vi "ULx Clear Task.vi"(0 "task in":refnum<k24>, 11 "error in":errorcluster) -> (15 "error out":errorcluster)   [LabVIEW 2020]
doc: "Clears the task. Before clearing, this VI stops the task, if necessary, and releases any resources the task reserved. You cannot use a task after you clear it unless you recreate the task."
uses:
  C:/Users/William/Documents/LV 2020 builds/LeaktestDAQ/Source-v33/ULx_LV.dll
  ULx_LV.dll
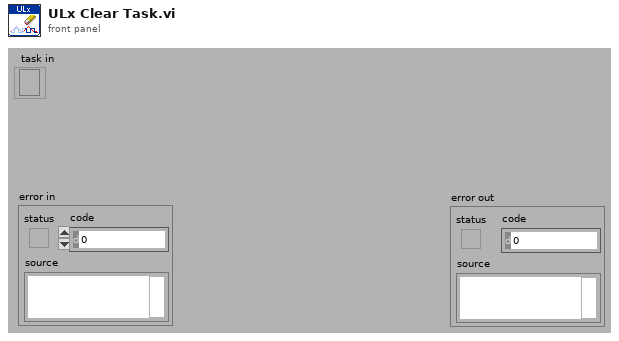
[diagram p1: front panel]
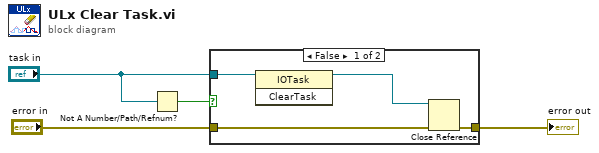
[diagram p0: block diagram]
diagram:
  n1 = Not A Number/Path/Refnum?(number/path/refnum="task in") -> (NaN/Path/Refnum?=w4:bool)
  n2 = case shown="False" w4 {
    tunnel: "task in" -> [w7 _]
    tunnel: [w8 w9] -> w1
    tunnel: "error in" -> [w5 w9]
    frame False {
      n3 = invoke class="IOTask" method="ClearTask"(reference=w7) -> (reference out=w6:refnum<k24>)  [unwired: 2 in, 2 out]
      n4 = Close Reference(reference=w6, error in (no error)=w5) -> (error out=w8:errorcluster)
    }
    frame True {
    }
  }
  "error out" <- w1
